vi "vms_monitorCommand_standby.vi"(8 "error in (no error)":errorcluster, 11 "command_standby_Ctl":T1) -> (0 "error out":errorcluster, 2 "function return":i32, 3 "command_standby_Ctl out":T1)   [LabVIEW 2016, in "SALLV_vms.lvlib"]
doc: "int vms_shm_monitorCommand_standbyLV(vms_command_standbyLV *command_standby_Ctl );"
uses:
  SALLV_vms.lvlib
  DataTypes/command_standby.ctl
  SALLV_vms.so
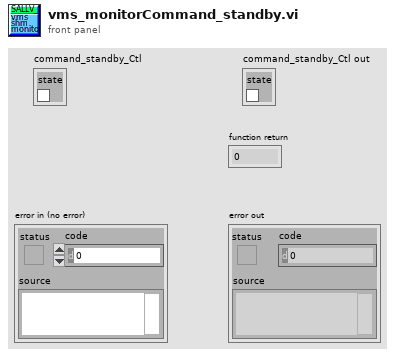
[diagram p1: front panel]
types:
  T1 = typedef "SALLV_vms.lvlib/command_standby.ctl" = cluster{"state":bool}
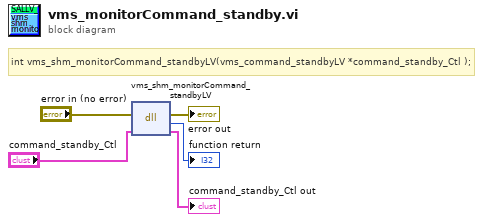
[diagram p0: block diagram]
diagram:
  # "int vms_shm_monitorCommand_standbyLV(vms_command_standbyLV *command_standby_Ctl );"
  n1 = dll-call lib="opt/CODE/SALLV_vms/SALLV_vms.*" fn="vms_shm_monitorCommand_standbyLV"(error in="error in (no error)", "command_standby_Ctl"="command_standby_Ctl") -> (error out=→"error out":errorcluster, →"function return":i32, "command_standby_Ctl"=→"command_standby_Ctl out":T1)  [unwired: 2 in, 1 out]
